vi "Misc Close Synchronization Objects.vi"(8 "error in (no error)":errorcluster, 11 "Cluster Reference":refnum<vi>) -> (0 "error out":errorcluster)   [LabVIEW 2011, in "Misc VIs.lvlib"]
uses:
  Misc VIs.lvlib
  Third Party/pcardinale/SubVIs/XML_Item_Type.ctl
  Third Party/pcardinale/pcardinale.lvlib
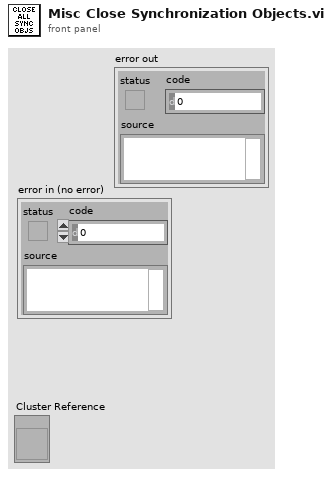
[diagram p1: front panel]
types:
  T1 = typedef "Third Party VIs.lvlib/pcardinale.lvlib/XML_Item_Type.ctl" = enum16{"String", "Start Tag", "Stop Tag", "Unified Tag"}
  T2 = typedef "Semaphore RefNum" = refnum<k1>
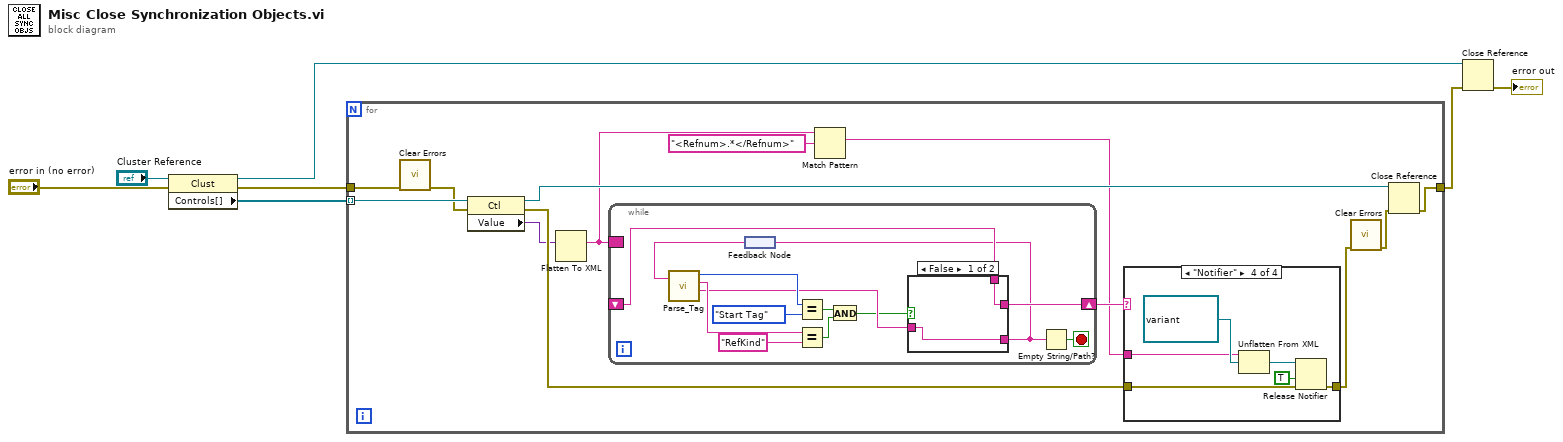
[diagram p0: block diagram]
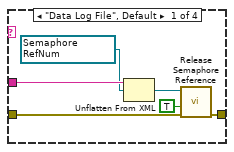
[diagram p2: hidden frame]
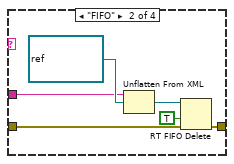
[diagram p3: hidden frame]
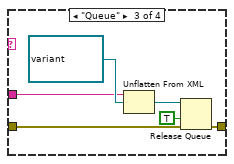
[diagram p4: hidden frame]
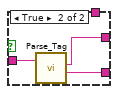
[diagram p5: hidden frame]
diagram:
  n1 = property class="Clust"(reference="Cluster Reference", error in="error in (no error)") -> (reference out=w1:refnum<vi>, error out=w3:errorcluster, "Controls[]"=w2:refnum<vi>[])
  n2 = for {
    tunnel: w2 -> [w20] mode=indexing
    tunnel: w3 -> [w12]
    tunnel: [w10] -> w7
    n3 = call <vilib>:"Clear Errors.vi"("error in (no error)"=w12) -> ("error out"=w11:errorcluster)  [unwired: 6 in]
    n4 = property class="Ctl"(reference=w20, error in=w11) -> (reference out=w19:refnum<vi>, error out=w17:errorcluster, "Value"=w15:variant)
    n5 = Flatten To XML(anything=w15) -> (xml string=w13:string)
    n6 = while {
      border: w13 -> [_]
      shift-right: [w51] -> w18
      shift-left: _ -> [w50]
      stop <- w57 stop-if-true
      n7 = feedback #1() -> (w56:string)
      n8 = call "Parse_Tag.vi"("String"=w56) -> ("Item Type"=w48:T1, "Item"=w49:string, "Remaining String"=w47:string)  [unwired: 2 in]
      n9 = Equal?(x=w48, y=XML_Item_Type."Start Tag") -> (x = y?=w53:bool)
      n10 = Equal?(x=w49, y="RefKind") -> (x = y?=w52:bool)
      n11 = And(x=w53, y=w52) -> (x .and. y?=w46:bool)
      n12 = case shown="False" w46 {
        tunnel: w47 -> [w59 w62]
        tunnel: [w59 w61] -> w45
        tunnel: [w58 w60] -> w51
        tunnel: w50 -> [w58 _]
        frame False {
        }
        frame True {
          n13 = call "Parse_Tag.vi"("String"=w62) -> ("Item"=w60:string, "Remaining String"=w61:string)  [unwired: 2 in, 1 out]
        }
      }
      n14 = feedback-in #1(w45) -> ()
      n15 = Empty String/Path?(string/path=w45) -> (empty?=w57:bool)
    }
    n16 = Match Pattern(string=w13, regular expression="<Refnum>.*</Refnum>") -> (match substring=w14:string)  [unwired: 1 in, 3 out]
    n17 = case shown="\"Notifier\"" w18 {
      tunnel: [w25 w31 w37 w43] -> w9
      tunnel: w17 -> [w24 w30 w36 w40]
      tunnel: w14 -> [w23 w28 w34 w39]
      frame "Data Log File", Default {
        w21 = T2 refnum items=["semaphore"] ("semaphore")
        n18 = Unflatten From XML(xml string=w23, type=w21) -> (value=w22:T2)  [unwired: 1 in, 1 out]
        n19 = call <vilib>:"Release Semaphore Reference.vi"("error in (no error)"=w24, "force destroy? (F)"=TRUE, "semaphore"=w22) -> ("error out"=w25:errorcluster)  [unwired: 7 in, 1 out]
      }
      frame "FIFO" {
        n20 = Unflatten From XML(xml string=w28, type=refnum<k33> refnum ("rt fifo")) -> (value=w27:refnum<k33>)  [unwired: 1 in, 1 out]
        n21 = RT FIFO Delete(0:w27, 2:TRUE ("force destroy? (F)"), 3:w30) -> (11:w31:errorcluster)
      }
      frame "Queue" {
        n22 = Unflatten From XML(xml string=w34, type=refnum<queue> refnum ("queue out")) -> (value=w33:refnum<queue>)  [unwired: 1 in, 1 out]
        n23 = Release Queue(queue=w33, force destroy? (F)=TRUE, error in (no error)=w36) -> (error out=w37:errorcluster)  [unwired: 2 out]
      }
      frame "Notifier" {
        n24 = Unflatten From XML(xml string=w39, type=refnum<notifier> refnum ("notifier out")) -> (value=w41:refnum<notifier>)  [unwired: 1 in, 1 out]
        n25 = Release Notifier(notifier=w41, force destroy? (F)=TRUE, error in (no error)=w40) -> (error out=w43:errorcluster)  [unwired: 2 out]
      }
    }
    n26 = call <vilib>:"Clear Errors.vi"("error in (no error)"=w9) -> ("error out"=w8:errorcluster)  [unwired: 6 in]
    n27 = Close Reference(reference=w19, error in (no error)=w8) -> (error out=w10:errorcluster)
  }
  n28 = Close Reference(reference=w1, error in (no error)=w7) -> (error out=→"error out":errorcluster)
